vi "Event Wait.vi"(8 "error in (no error)":errorcluster, 11 "Event DVR in":refnum<data-value>) -> (0 "error out":errorcluster, 3 "Event DVR out":refnum<data-value>)   [LabVIEW 2010, in "MDSplus.lvlib"]
doc: "Return data received last."
uses:
  <vilib>/MDSplus/Library/MDSplus.lvlib
  <vilib>/MDSplus/Classes/Event_Class/Event.lvclass
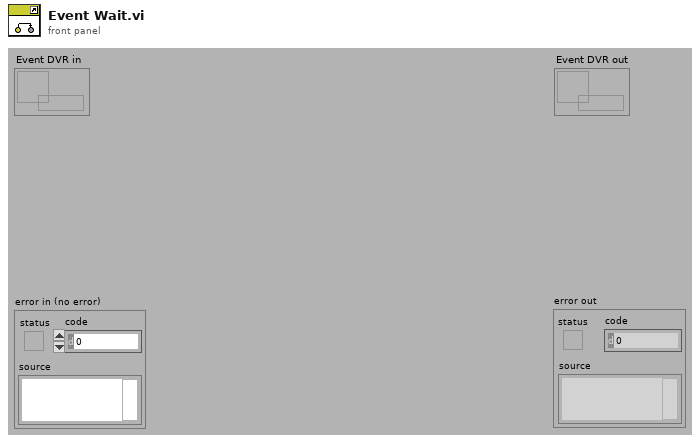
[diagram p1: front panel]
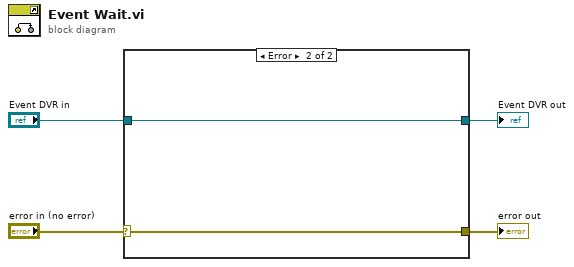
[diagram p0: block diagram]
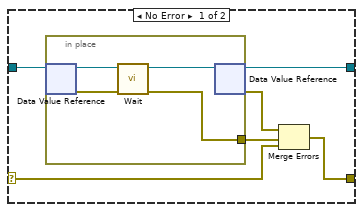
[diagram p2: hidden frame]
diagram:
  n1 = case shown="Error" "error in (no error)" {
    selector: "error in (no error)" -> [w9 w16]
    tunnel: "Event DVR in" -> [w10 w15]
    tunnel: [w6 w16] -> w4
    tunnel: [w7 w15] -> w1
    frame No Error {
      n2 = in-place {
        in-place-border: [w11] -> w5
        n3 = in-place-dvr #1(w10) -> (w14:refnum<class "Event.lvclass">, w13:errorcluster)
        n4 = call-dynamic "Wait.vi"("error in (no error)"=w13, "Event in"=w14) -> ("error out"=w11:errorcluster, "Event out"=w12:refnum<class "Event.lvclass">)  [unwired: 8 in]
        n5 = in-place-dvr #1(w12) -> (w7:refnum<data-value>, w8:errorcluster)
      }
      n6 = Merge Errors(w8, w5, w9) -> (w6:errorcluster)
    }
    frame Error {
    }
  }
  "error out" <- w4
  "Event DVR out" <- w1
